vi "module check.vi"(2 "error in":errorcluster, 4 "Value":dbl) -> (0 "error constant":errorcluster, 1 "Value out":dbl)   [LabVIEW 2016]
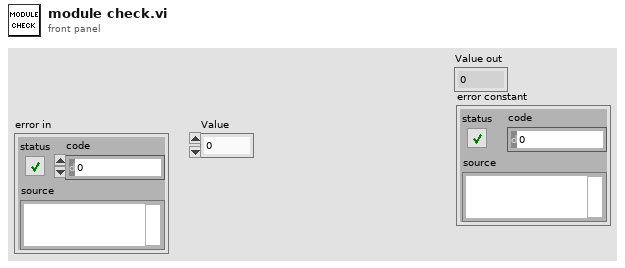
[diagram p1: front panel]
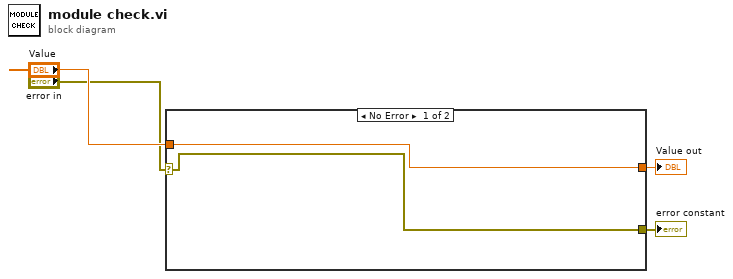
[diagram p0: block diagram]
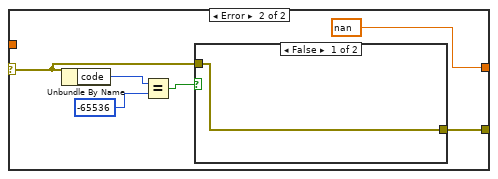
[diagram p2: hidden frame]
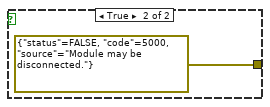
[diagram p3: hidden frame]
diagram:
  n1 = case shown="No Error" "error in" {
    selector: "error in" -> [w6 w9]
    tunnel: "Value" -> [w5 _]
    tunnel: [w5 nan] -> w2
    tunnel: [w6 w7] -> w1
    frame No Error {
    }
    frame Error {
      n2 = Unbundle By Name(w9) -> ("code"=w12:i32)
      n3 = Equal?(x=w12, y=-65536) -> (x = y?=w10:bool)
      n4 = case shown="False" w10 {
        tunnel: [w13 errorcluster {"status"=FALSE, "code"=5000, "source"="Module may be disconnected."} ("error constant")] -> w7
        tunnel: w9 -> [w13 _]
        frame False {
        }
        frame True {
        }
      }
    }
  }
  "Value out" <- w2
  "error constant" <- w1
